vi "destroy.vi"(8 "error in (no error)":errorcluster, 11 "timer":refnum<class "rytimer.lvclass">) -> (0 "error out":errorcluster)   [LabVIEW 2017, in "rytimer.lvclass"]
uses:
  rytimer.lvclass
  rytimer.lvclass/rytimer.ctl
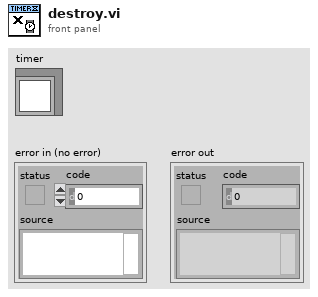
[diagram p1: front panel]
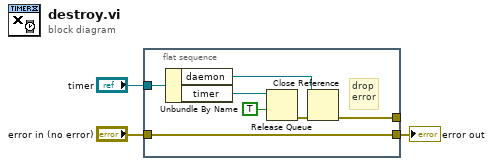
[diagram p0: block diagram]
diagram:
  n1 = flat-sequence {
    tunnel: "timer" -> [w10]
    tunnel: [w8] -> w2
    tunnel: "error in (no error)" -> [w8]
    tunnel: [w4] -> _
    frame #0 {
      # "drop\nerror"
      n2 = Unbundle By Name(w10) -> ("daemon"=w5:refnum<vi>, "timer"=w9:refnum<queue>)
      n3 = Release Queue(queue=w9, force destroy? (F)=TRUE) -> (error out=w6:errorcluster)  [unwired: 1 in, 2 out]
      n4 = Close Reference(reference=w5, error in (no error)=w6) -> (error out=w4:errorcluster)
    }
  }
  "error out" <- w2
